vi "XYStage.MoveAbsolute (units).vi"(7 "Wait Timeout, ms (60000)":i32=60000, 8 "error in (no error)":errorcluster, 10 "Units":T1, 11 "XYStage.KIM101 in":refnum<class "XYStage.KIM101.lvclass">) -> (0 "error out":errorcluster, 3 "XYStage.KIM101 out":refnum<class "XYStage.KIM101.lvclass">)   [LabVIEW 2017, in "XYStage.KIM101.lvclass"]
uses:
  XYStage.KIM101.lvclass
  XYStage/Typedefs/Coordinates.Units--Cluster.ctl
  D:/upwork/Laser Measurement Tool/Laser/project/data/Thorlabs.MotionControl.KCube.InertialMotorCLI.dll
  data/Thorlabs.MotionControl.KCube.InertialMotorCLI.dll
  XYStage/XYStage.lvclass
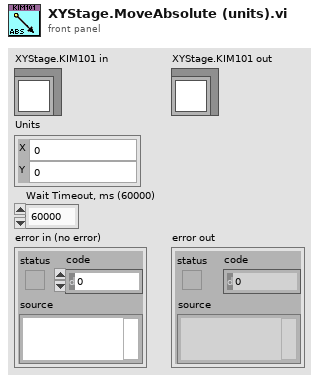
[diagram p1: front panel]
types:
  T1 = typedef "XYStage.lvclass/Coordinates.Units--Cluster.ctl" = cluster{"X":dbl, "Y":dbl}
  T2 = typedef "XYStage.KIM101.lvclass/Resource--Cluster.ctl" = cluster{"KCubeInertialMotorControl":refnum<k24>, "Device":refnum<k24>, "X Axis Channel":i32, "Y Axis Channel":i32}
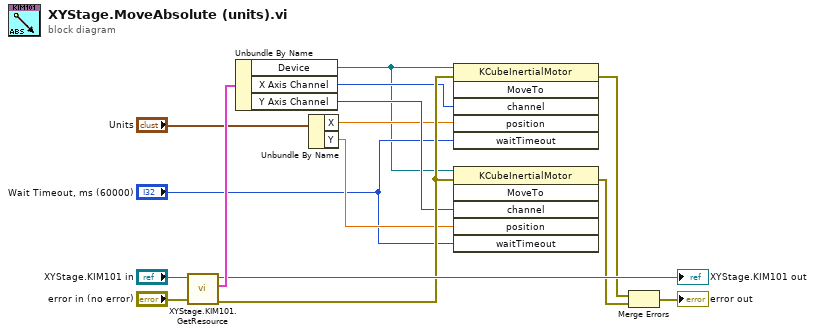
[diagram p0: block diagram]
diagram:
  n1 = call "XYStage.KIM101.GetResource.vi"("error in (no error)"="error in (no error)", "XYStage.KIM101 in"="XYStage.KIM101 in") -> ("error out"=w11:errorcluster, "Resource"=w13:T2, "XYStage.KIM101 out"=→"XYStage.KIM101 out":refnum<class "XYStage.KIM101.lvclass">)  [unwired: 7 in]
  n2 = Unbundle By Name(w13) -> ("Device"=w1:refnum<k24>, "X Axis Channel"=w7:i32, "Y Axis Channel"=w6:i32)
  n3 = Unbundle By Name("Units") -> ("X"=w4:dbl, "Y"=w3:dbl)
  n4 = invoke class="KCubeInertialMotor" method="MoveTo"(reference=w1, error in=w11, "channel"=w7, "position"=w4, "waitTimeout"="Wait Timeout, ms (60000)") -> (error out=w8:errorcluster)  [unwired: 1 in, 5 out]
  n5 = invoke class="KCubeInertialMotor" method="MoveTo"(reference=w1, error in=w11, "channel"=w6, "position"=w3, "waitTimeout"="Wait Timeout, ms (60000)") -> (error out=w9:errorcluster)  [unwired: 1 in, 5 out]
  n6 = Merge Errors(w8, w9) -> (→"error out":errorcluster)
